vi "Test-Motors with Brake-Percent.vi"() -> ()   [LabVIEW 2014, in "Comp Motors with Brake.lvlib"]
uses:
  Comp Motors with Brake.lvlib
  Robot Actor Framework/Trace/Trace Controller Class/Config.ctl
  Comp Motors with Encoders/Comp Motors with Encoders Class/Motor Controller Config.ctl
  Robot/Motor with Encoders/Motors with Encoders Class/Motors with Encoders Config.ctl
  Comp Motors with Encoders/Comp Motors with Encoders Class/Encoder Config.ctl
  Comp Motors with Brake Class/Comp Motors with Brake Config.ctl
  <vilib>/Rock Robotics/WPI/Solenoid/WPI_SolenoidChannel.ctl
  Comp Trace Controller/Comp Trace Controller Class/Comp Trace Controller.lvclass
  Comp Pressure/Comp Pressure Class/Comp Pressure.lvclass
  Comp Motors with Brake Class/Comp Motors with Brake.lvclass
  <vilib>/Rock Robotics/WPI/DriverStation/WPI_DriverStationRobotMode2.ctl
  Robot/Motor with Encoders/Motors with Encoders Messages/Set Rate (Percent) Msg/Set Rate (Percent) Msg.lvclass/Set Rate (Percent) Msg.ctl
  <vilib>/ActorFramework/Message Enqueuer/Message Enqueuer.lvclass/Message Enqueuer.ctl
  <vilib>/ActorFramework/Message Enqueuer/Enqueue.vi
  <vilib>/ActorFramework/Message Priority Queue/Priority Enqueue.vi
  Robot/Motor with Encoders/Motors with Encoders Messages/Set Rate (Percent) Msg/Set Rate (Percent) Msg.lvclass
  <vilib>/ActorFramework/Stop Msg/Stop Msg.lvclass
  <vilib>/ActorFramework/Actor/Actor.lvclass
  Robot Actor Framework/Trace/Trace Controller Class/Trace Controller.lvclass
  Comp Motors with Encoders/Comp Motors with Encoders Class/Comp Motors with Encoders.lvclass
  Robot/Motor with Encoders/Motors with Encoders Class/Motors with Encoders.lvclass
panel:
  in  "Comp Motors with Brake Config":T1={"Brake Channel"=enum."Solenoid 6", "Pneumatics CAN ID"=3}
  in  "Test Loop":u32=75
  in  "Encoder Config":T3={"P"=1.0, "D"=0.0, "F"=0.01, "I"=0.01, "Reverse Feedback Sensor"=FALSE, "Encoder Codes Per Rev"=256}
  out "Enable Tele":bool caption="Enabled Teleop"
  in  "Stop Test Loop 1":bool=TRUE
  in  "Finish Test":bool=TRUE
  in  "Start Test":bool=TRUE
  in  "Rate (Percent)":dbl(slide) scale=-1.0..1.0
  in  "Motos with Encoder Config":T4={"Counts  Per Revolution"=256, "Invert Encoder Direction"=FALSE, "Diameter of Revolution"=6.0, "Max RPM"=1500.0, "Encoder Control"=TRUE}
  in  "Slave Motor Controller Configs":T5[](array[typedef])
  in  "Master Motor Controller Config":T5={"Device Number"=7, "Invert Motor"=FALSE}
  in  "Trace Controller Config":T6={"Folder Pattern"="/media/sd%s1", "Starting Letter Position"=1, "Min Free Space (MB)"=50.0, "Max Folders to Check"=10, "Trace Level"=enum."Debug"} {"Min Free Space (MB)" format="%#_13g"}
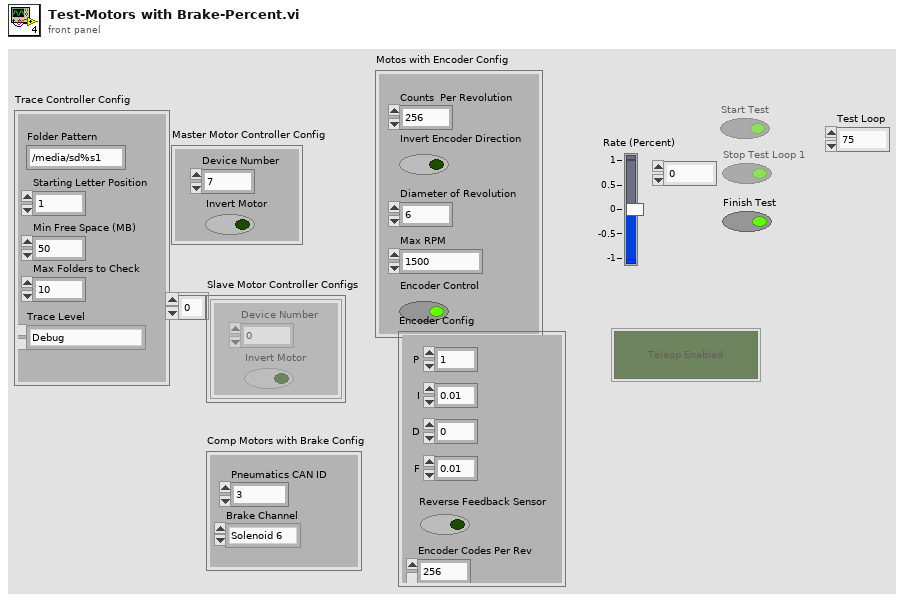
[diagram p1: front panel]
types:
  T1 = typedef "Comp Motors with Brake.lvlib/Comp Motors with Brake.lvclass/Comp Motors with Brake Config.ctl" = cluster{"Brake Channel":T2, "Pneumatics CAN ID":u8}
  T2 = typedef "WPI_SolenoidChannel.ctl" = enum8{"Solenoid 0", "Solenoid 1", "Solenoid 2", "Solenoid 3", "Solenoid 4", "Solenoid 5", "Solenoid 6", "Solenoid 7", "Invalid"}
  T3 = typedef "Comp Motors with Encoders.lvlib/Comp Motors with Encoders.lvclass/Encoder Config.ctl" = cluster{"P":dbl, "D":dbl, "F":dbl, "I":dbl, "Reverse Feedback Sensor":bool, "Encoder Codes Per Rev":u16}
  T4 = typedef "Motors with Encoders.lvlib/Motors with Encoders.lvclass/Motors with Encoders Config.ctl" = cluster{"Counts  Per Revolution":u32, "Invert Encoder Direction":bool, "Diameter of Revolution":dbl, "Max RPM":dbl, "Encoder Control":bool}
  T5 = typedef "Comp Motors with Encoders.lvlib/Comp Motors with Encoders.lvclass/Motor Controller Config.ctl" = cluster{"Device Number":u8, "Invert Motor":bool}
  T6 = typedef "Robot Actor Framework.lvlib/Trace.lvlib/Trace Controller.lvclass/Config.ctl" = cluster{"Folder Pattern":string, "Starting Letter Position":i32, "Min Free Space (MB)":dbl, "Max Folders to Check":u32, "Trace Level":enum16{"Critical", "Error", "Warning", "Informational", "Debug"}}
  T7 = enum16{"Critical", "Error", "Warning", "Informational", "Debug"}
  T8 = enum8{"Enabled", "Disabled", "Disabled and Grayed Out"}
  T9 = typedef "WPI_DriverStationRobotMode2.ctl" = enum16{"Autonomous Disabled", "Autonomous Enabled", "Teleop Disabled", "Teleop Enabled", "Disconnected", "Finish", "Test Disabled", "Test Enabled", "Emergency Stopped"}
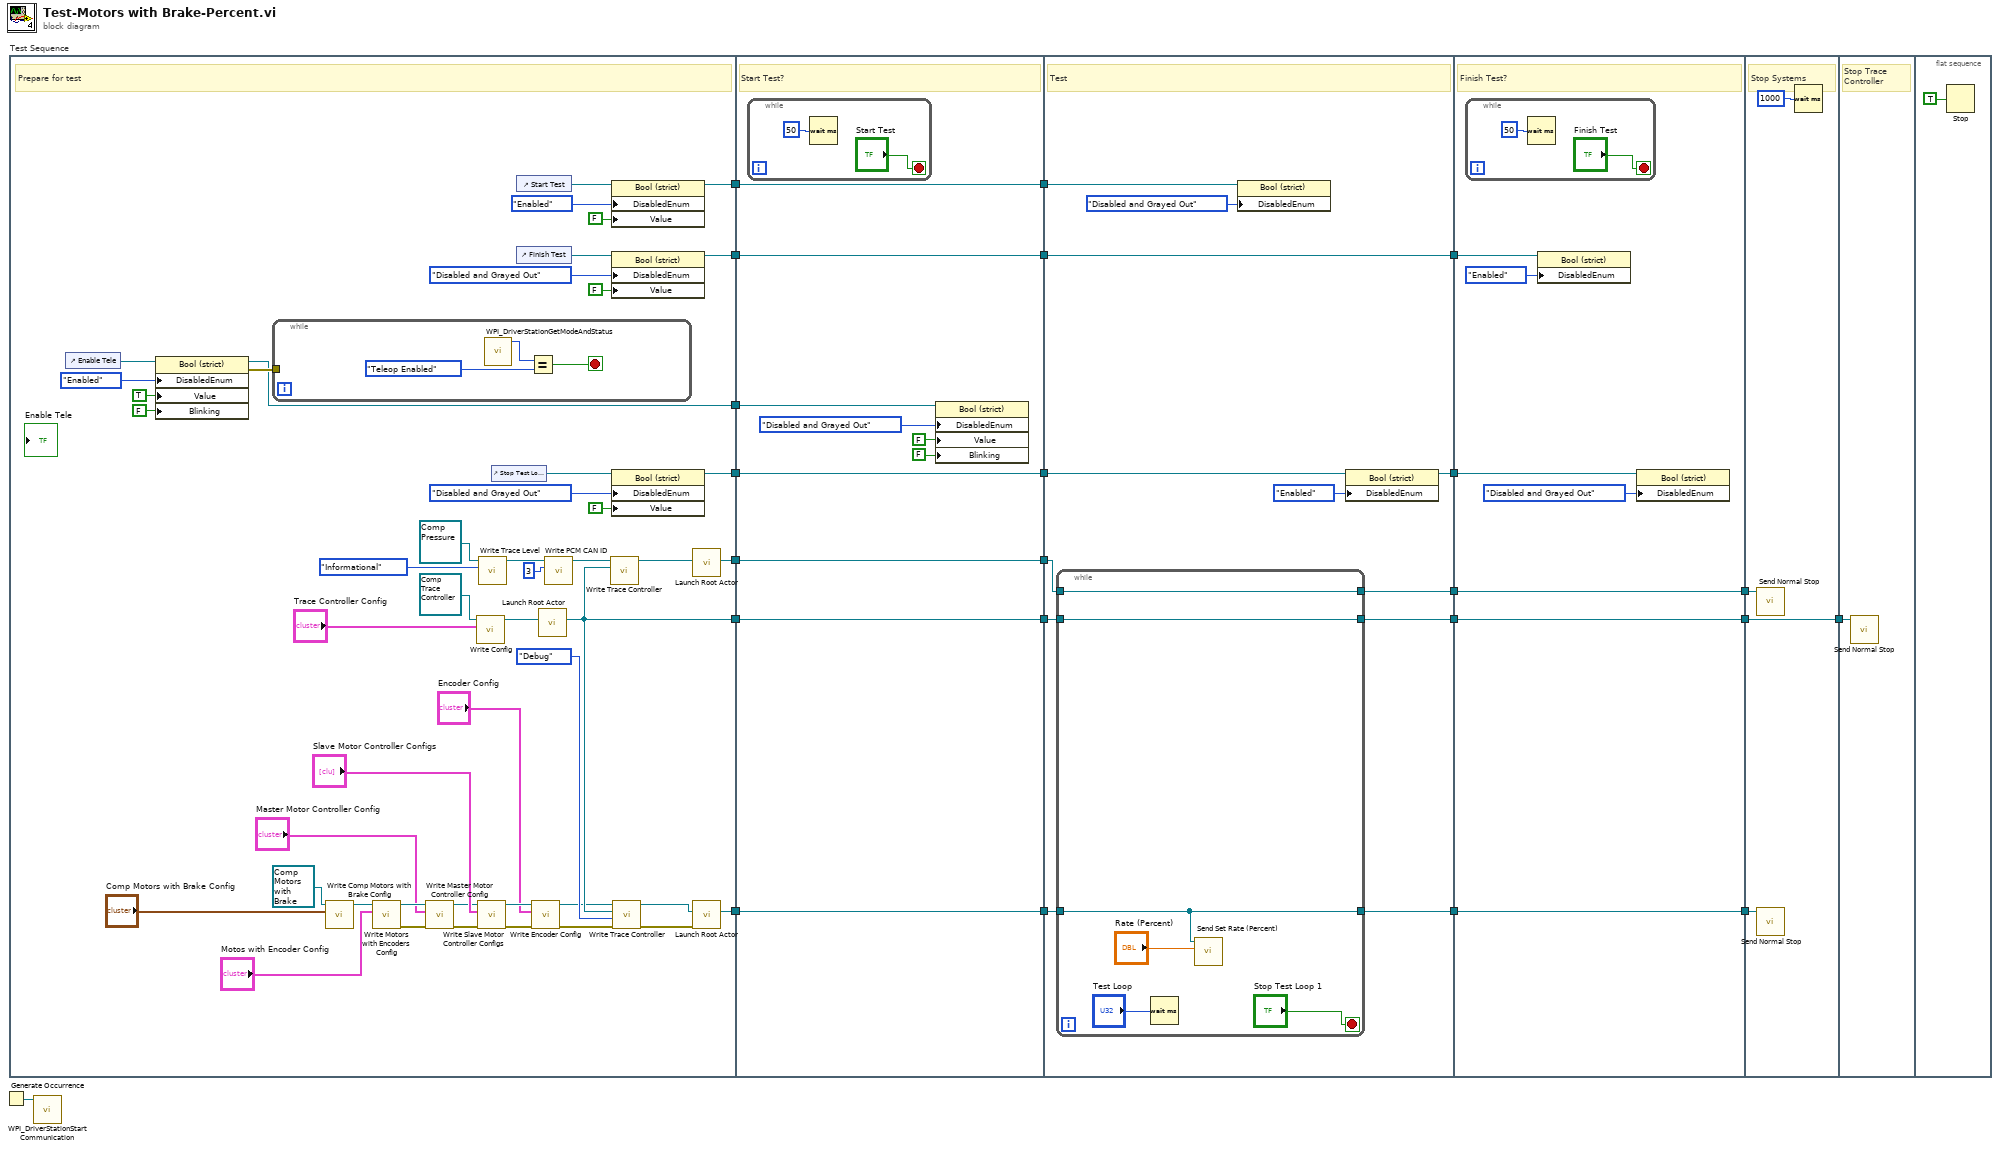
[diagram p0: block diagram]
diagram:
  n1 = Generate Occurrence() -> (w23:refnum<k4>)
  n2 = flat-sequence "Test Sequence" {
    tunnel: [w54] -> w12
    tunnel: [w56] -> w11
    tunnel: [w55] -> w10
    tunnel: [w44] -> w9
    tunnel: [w43] -> w7
    tunnel: [w42] -> w2
    tunnel: [w36] -> w1
    tunnel: [w84] -> w15
    tunnel: [w83] -> w14
    tunnel: [w82] -> w13
    tunnel: w12 -> [w84]
    tunnel: w11 -> [w83]
    tunnel: w10 -> [w82]
    tunnel: w9 -> [w81]
    tunnel: [w81] -> w8
    tunnel: w7 -> [w80]
    tunnel: [w80] -> w6
    tunnel: [w79] -> w3
    tunnel: w2 -> [w79]
    tunnel: w1 -> [w78]
    tunnel: [w93] -> w18
    tunnel: [w95] -> w17
    tunnel: [w94] -> w16
    tunnel: w15 -> [w98]
    tunnel: w14 -> [w96]
    tunnel: w13 -> [w97]
    tunnel: w8 -> [w92]
    tunnel: w6 -> [w90]
    tunnel: [w88] -> w5
    tunnel: [w87] -> w4
    tunnel: w3 -> [w87]
    tunnel: [w111] -> w21
    tunnel: [w110] -> w20
    tunnel: [w109] -> w19
    tunnel: w18 -> [w111]
    tunnel: w17 -> [w110]
    tunnel: w16 -> [w109]
    tunnel: w5 -> [w108]
    tunnel: w4 -> [w105]
    tunnel: [w117] -> w22
    tunnel: w21 -> [w117]
    tunnel: w20 -> [w116]
    tunnel: w19 -> [w114]
    tunnel: w22 -> [w118]
    frame #0 {
      # "Prepare for test"
      n3 = control-ref of="Enable Tele"() -> (w41:refnum<vi>)
      n4 = property class="Bool (strict)"(reference=w41, "DisabledEnum"=T8."Enabled" ("Disabled"), "Value"=TRUE, "Blinking"=FALSE) -> (reference out=w36:refnum<vi>, error out=w38:errorcluster)  [unwired: 1 in]
      n5 = while {
        tunnel: w38 -> [_]
        stop <- w72 stop-if-true
        n6 = call <vilib>:"WPI_DriverStationGetModeAndStatus.vi"() -> ("Robot Mode"=w74:T9)  [unwired: 10 in, 1 out]
        n7 = Equal?(x=w74, y=WPI_DriverStationRobotMode2."Teleop Enabled") -> (x = y?=w72:bool)
      }
      n8 = call-dynamic "Write Comp Motors with Brake Config.vi"("Comp Motors with Brake Config"="Comp Motors with Brake Config", "Comp Motors with Brake in"=refnum<class "Comp Motors with Brake.lvclass"> refnum ("Comp Motors with Brake.lvlib:Comp Motors with Brake.lvclass")) -> ("Comp Motors with Brake out"=w25:refnum<class "Comp Motors with Brake.lvclass">)  [unwired: 8 in, 1 out]
      n9 = call-dynamic "Write Motors with Encoders Config.vi"("Motors with Encoders Config"="Motos with Encoder Config", "Motors with Encoders in"=w25) -> ("error out"=w63:errorcluster, "Motors with Encoders out"=w29:refnum<class "Comp Motors with Brake.lvclass">)  [unwired: 8 in]
      n10 = call-dynamic "Write Master Motor Controller Config.vi"("error in (no error)"=w63, "Master Motor Controller Config"="Master Motor Controller Config", "Comp Motors with Encoders in"=w29) -> ("error out"=w64:errorcluster, "Comp Motors with Encoders out"=w60:refnum<class "Comp Motors with Brake.lvclass">)  [unwired: 7 in]
      n11 = call-dynamic "Write Config.vi"("Config"="Trace Controller Config", "Trace Controller in"=refnum<class "Comp Trace Controller.lvclass"> refnum ("Comp Trace Controller.lvlib:Comp Trace Controller.lvclass")) -> ("Trace Controller out"=w59:refnum<class "Comp Trace Controller.lvclass">)  [unwired: 8 in, 1 out]
      n12 = call-dynamic "Write Slave Motor Controller Configs.vi"("error in (no error)"=w64, "Slave Motor Controller Configs"="Slave Motor Controller Configs", "Comp Motors with Encoders in"=w60) -> ("error out"=w34:errorcluster, "Comp Motors with Encoders out"=w35:refnum<class "Comp Motors with Brake.lvclass">)  [unwired: 7 in]
      n13 = call-dynamic "Write Trace Level.vi"("Trace Level"=T7."Informational", "System Actor in"=refnum<class "Comp Pressure.lvclass"> refnum ("Comp Pressure.lvlib:Comp Pressure.lvclass")) -> ("System Actor out"=w69:refnum<class "Comp Pressure.lvclass">)  [unwired: 8 in, 1 out]
      n14 = control-ref of="Stop Test Loop 1"() -> (w48:refnum<vi>)
      n15 = control-ref of="Start Test"() -> (w53:refnum<vi>)
      n16 = control-ref of="Finish Test"() -> (w47:refnum<vi>)
      n17 = call-dynamic "Write Encoder Config.vi"("error in (no error)"=w34, "Encoder Config"="Encoder Config", "Comp Motors with Encoders in"=w35) -> ("error out"=w33:errorcluster, "Comp Motors with Encoders out"=w27:refnum<class "Comp Motors with Brake.lvclass">)  [unwired: 7 in]
      n18 = call <vilib>:"Launch Root Actor.vi"("Actor"=w59) -> ("Actor's Enqueuer"=w55:refnum<class "Message Enqueuer.lvclass">)  [unwired: 9 in, 1 out]
      n19 = call-dynamic "Write PCM CAN ID.vi"("PCM CAN ID"=u8 3, "Comp Pressure in"=w69) -> ("Comp Pressure out"=w70:refnum<class "Comp Pressure.lvclass">)  [unwired: 8 in, 1 out]
      n20 = call-dynamic "Write Trace Controller.vi"("Trace Controller"=w55, "System Actor in"=w70) -> ("System Actor out"=w71:refnum<class "Comp Pressure.lvclass">)  [unwired: 8 in, 1 out]
      n21 = property class="Bool (strict)"(reference=w53, "DisabledEnum"=T8."Enabled" ("Disabled"), "Value"=FALSE) -> (reference out=w44:refnum<vi>)  [unwired: 1 in, 1 out]
      n22 = property class="Bool (strict)"(reference=w47, "DisabledEnum"=T8."Disabled and Grayed Out" ("Disabled"), "Value"=FALSE) -> (reference out=w42:refnum<vi>)  [unwired: 1 in, 1 out]
      n23 = property class="Bool (strict)"(reference=w48, "DisabledEnum"=T8."Disabled and Grayed Out" ("Disabled"), "Value"=FALSE) -> (reference out=w43:refnum<vi>)  [unwired: 1 in, 1 out]
      n24 = call-dynamic "Write Trace Controller.vi"("error in (no error)"=w33, "Trace Level"=T7."Debug", "Trace Controller"=w55, "System Actor in"=w27) -> ("error out"=w66:errorcluster, "System Actor out"=w65:refnum<class "Comp Motors with Brake.lvclass">)  [unwired: 6 in]
      n25 = call <vilib>:"Launch Root Actor.vi"("Actor"=w71) -> ("Actor's Enqueuer"=w56:refnum<class "Message Enqueuer.lvclass">)  [unwired: 9 in, 1 out]
      n26 = call <vilib>:"Launch Root Actor.vi"("error in (no error)"=w66, "Actor"=w65) -> ("Actor's Enqueuer"=w54:refnum<class "Message Enqueuer.lvclass">)  [unwired: 8 in, 1 out]
    }
    frame #1 {
      # "Start Test?"
      n27 = while {
        stop <- "Start Test" stop-if-true
        n28 = Wait (ms)(milliseconds to wait=u32 50) -> ()  [unwired: 1 out]
      }
      n29 = property class="Bool (strict)"(reference=w78, "DisabledEnum"=T8."Disabled and Grayed Out" ("Disabled"), "Value"=FALSE, "Blinking"=FALSE) -> ()  [unwired: 1 in, 2 out]
    }
    frame #2 {
      # "Test"
      n30 = while {
        tunnel: w97 -> [w103]
        tunnel: [w103] -> w93
        tunnel: w98 -> [w100]
        tunnel: [w100] -> w95
        tunnel: w96 -> [w102]
        tunnel: [w102] -> w94
        stop <- "Stop Test Loop 1" stop-if-true
        n31 = Wait (ms)(milliseconds to wait="Test Loop") -> ()  [unwired: 1 out]
        n32 = call "Send Set Rate (Percent).vi"("Rate (Percentage)"="Rate (Percent)", "Message Enqueuer"=w100) -> ()  [unwired: 8 in, 2 out]
      }
      n33 = property class="Bool (strict)"(reference=w92, "DisabledEnum"=T8."Disabled and Grayed Out" ("Disabled")) -> ()  [unwired: 1 in, 2 out]
      n34 = property class="Bool (strict)"(reference=w90, "DisabledEnum"=T8."Enabled" ("Disabled")) -> (reference out=w88:refnum<vi>)  [unwired: 1 in, 1 out]
    }
    frame #3 {
      # "Finish Test?"
      n35 = while {
        stop <- "Finish Test" stop-if-true
        n36 = Wait (ms)(milliseconds to wait=u32 50) -> ()  [unwired: 1 out]
      }
      n37 = property class="Bool (strict)"(reference=w105, "DisabledEnum"=T8."Enabled" ("Disabled")) -> ()  [unwired: 1 in, 2 out]
      n38 = property class="Bool (strict)"(reference=w108, "DisabledEnum"=T8."Disabled and Grayed Out" ("Disabled")) -> ()  [unwired: 1 in, 2 out]
    }
    frame #4 {
      # "Stop Systems"
      n39 = call <vilib>:"Send Normal Stop.vi"("Message Enqueuer"=w114) -> ()  [unwired: 10 in, 1 out]
      n40 = call <vilib>:"Send Normal Stop.vi"("Message Enqueuer"=w116) -> ()  [unwired: 10 in, 1 out]
      n41 = Wait (ms)(milliseconds to wait=u32 1000) -> ()  [unwired: 1 out]
    }
    frame #5 {
      # "Stop Trace Controller"
      n42 = call <vilib>:"Send Normal Stop.vi"("Message Enqueuer"=w118) -> ()  [unwired: 10 in, 1 out]
    }
    frame #6 {
      n43 = Stop(stop? (T)=TRUE) -> ()
    }
  }
  n44 = call <vilib>:"WPI_DriverStationStart Communication.vi"("occurrence"=w23) -> ()  [unwired: 1 in, 10 out]
